vi "array serach test.vi"() -> ()   [LabVIEW 2010]
panel:
  in  "String":string="string"
  out "Numeric":dbl
  in  "Array":string[](array[string])
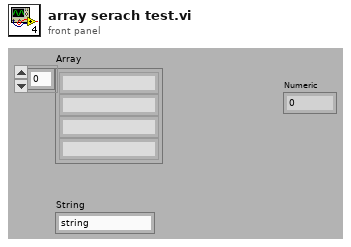
[diagram p1: front panel]
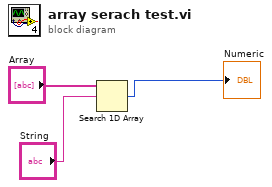
[diagram p0: block diagram]
diagram:
  n1 = Search 1D Array(1D array="Array", element="String") -> (index of element=→"Numeric":i32)  [unwired: 1 in]
